vi "Close Handle.vi"(8 "error in":errorcluster, 11 "Read Event in":refnum<class "Read Event.lvclass">) -> (0 "error out":errorcluster, 3 "Read Event out":refnum<class "Read Event.lvclass">)   [LabVIEW 2019, in "PCANBasic.lvlib" / "Read Event.lvclass"]
doc: "If the function succeeds, the return value is a handle to the event object."
uses:
  Read Event.lvclass
  Read Event.lvclass/Read Event.ctl
  Event Handle.ctl
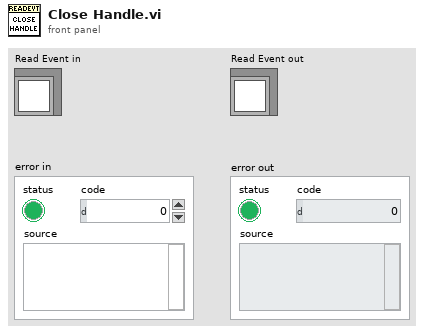
[diagram p1: front panel]
types:
  T1 = typedef "PCANBasic.lvlib/Read Event.lvclass/Event Handle.ctl" = u64
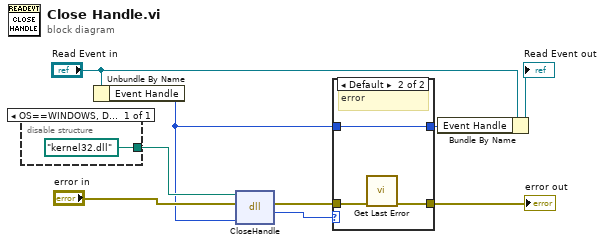
[diagram p0: block diagram]
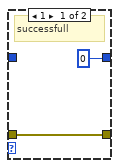
[diagram p2: hidden frame]
diagram:
  n1 = disable-structure shown="OS==WINDOWS, Default" {
    disable-tunnel: [path "kernel32.dll" ("path in")] -> w9
    frame condition #0 (active) {
    }
  }
  n2 = Unbundle By Name("Read Event in") -> ("Event Handle"=w1:T1)
  n3 = dll-call lib="?" fn="CloseHandle"(path in=w9, error in="error in", "hdlEvent"=w1) -> (error out=w7:errorcluster, "status"=w5:i32)  [unwired: 2 in, 1 out]
  n4 = case "success?" shown="Default" w5 {
    tunnel: w7 -> [w12 w15]
    tunnel: [w12 w14] -> w6
    tunnel: [T1 0 ("Event Handle") w13] -> w2
    tunnel: w1 -> [_ w13]
    frame 1 {
      # "successfull"
    }
    frame Default {
      # "error"
      n5 = call "Get Last Error.vi"("error in"=w15) -> ("error out"=w14:errorcluster)  [unwired: 10 in]
    }
  }
  "error out" <- w6
  n6 = Bundle By Name(cluster="Read Event in", "Event Handle"=w2) -> (→"Read Event out":refnum<class "Read Event.lvclass">)
